vi "get_data_from_sensors.vi"() -> ()   [LabVIEW 2015]
uses:
  <vilib>/Analysis/baseanly.llb/Mean (DBL).vi
  <vilib>/ErrorRing/Error Ring.xnode
  <vilib>/Analysis/NI_AALBase.lvlib
panel:
  out "mean thermometer":dbl format="%0.2f"
  out "mean potentiometer":dbl format="%0.2f"
  out "min value potentiometer":sgl
  out "max value potentiometer":sgl
  out "min value thermometer":sgl
  out "max value thermometer":sgl
  out "Thermometer values":sgl[](array[numeric])
  out "Potentiometer values":sgl[](array[numeric])
  out "error out 3":errorcluster
  out "error out 2":errorcluster
  out "error out":errorcluster
  in  "stop":bool
  out "timed out?\nBattery Voltage\nPotentiometer":bool
  out "timed out?\nLink Quality\nPotentiometer":bool
  out "timed out?\nBattery Voltage\nTemperature":bool
  out "timed out?\nLink Quality\nTemperature":bool
  out "Link Quality\nTemperature (3212)":sgl
  out "Battery Voltage \nTemperature (3212)":sgl
  out "Link Quality\nPotentiometer (3202)":sgl
  out "Battery Voltage\nPotentiometer (3202)":sgl
  out "Waveform Chart":dbl(graph)
  out "Numeric":dbl
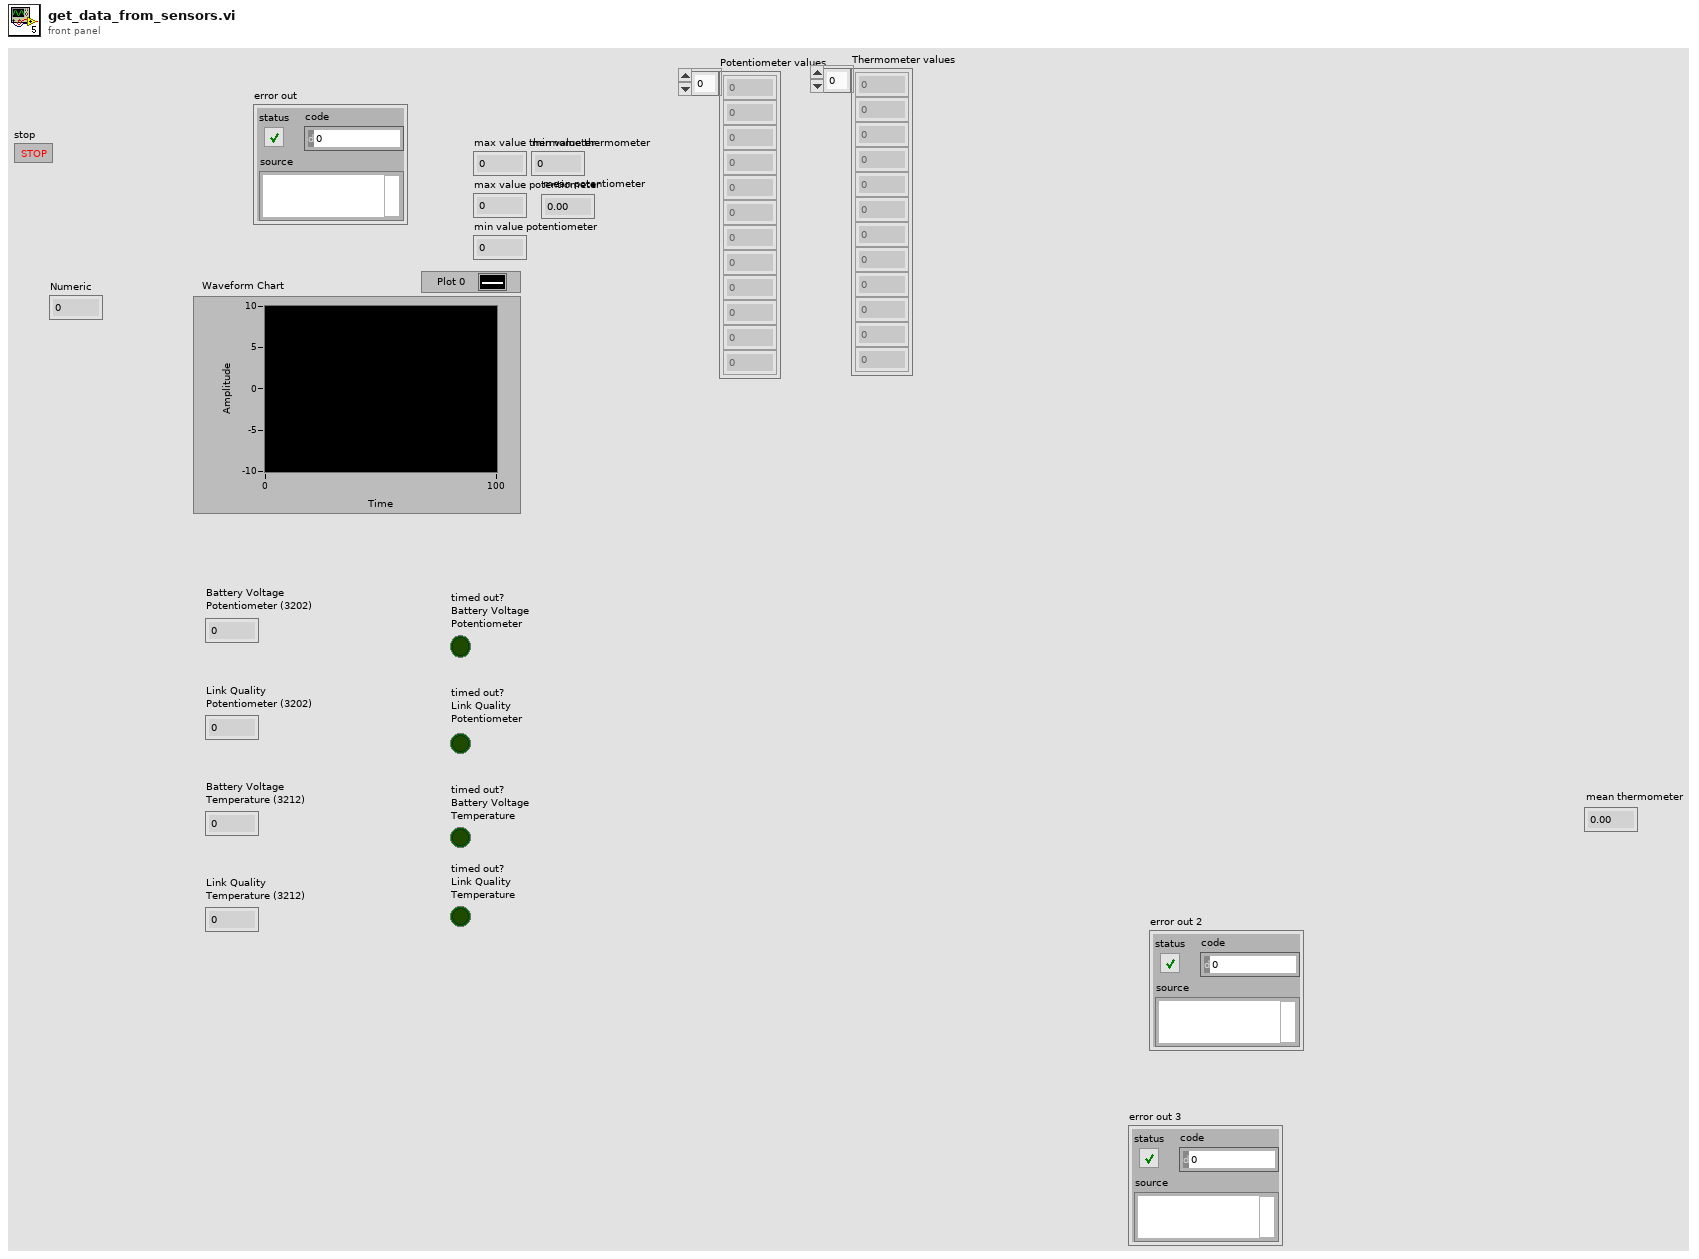
[diagram p1: front panel]
types:
  T1 = enum16{"open", "replace", "create", "open or create", "replace or create", "replace or create with confirmation"}
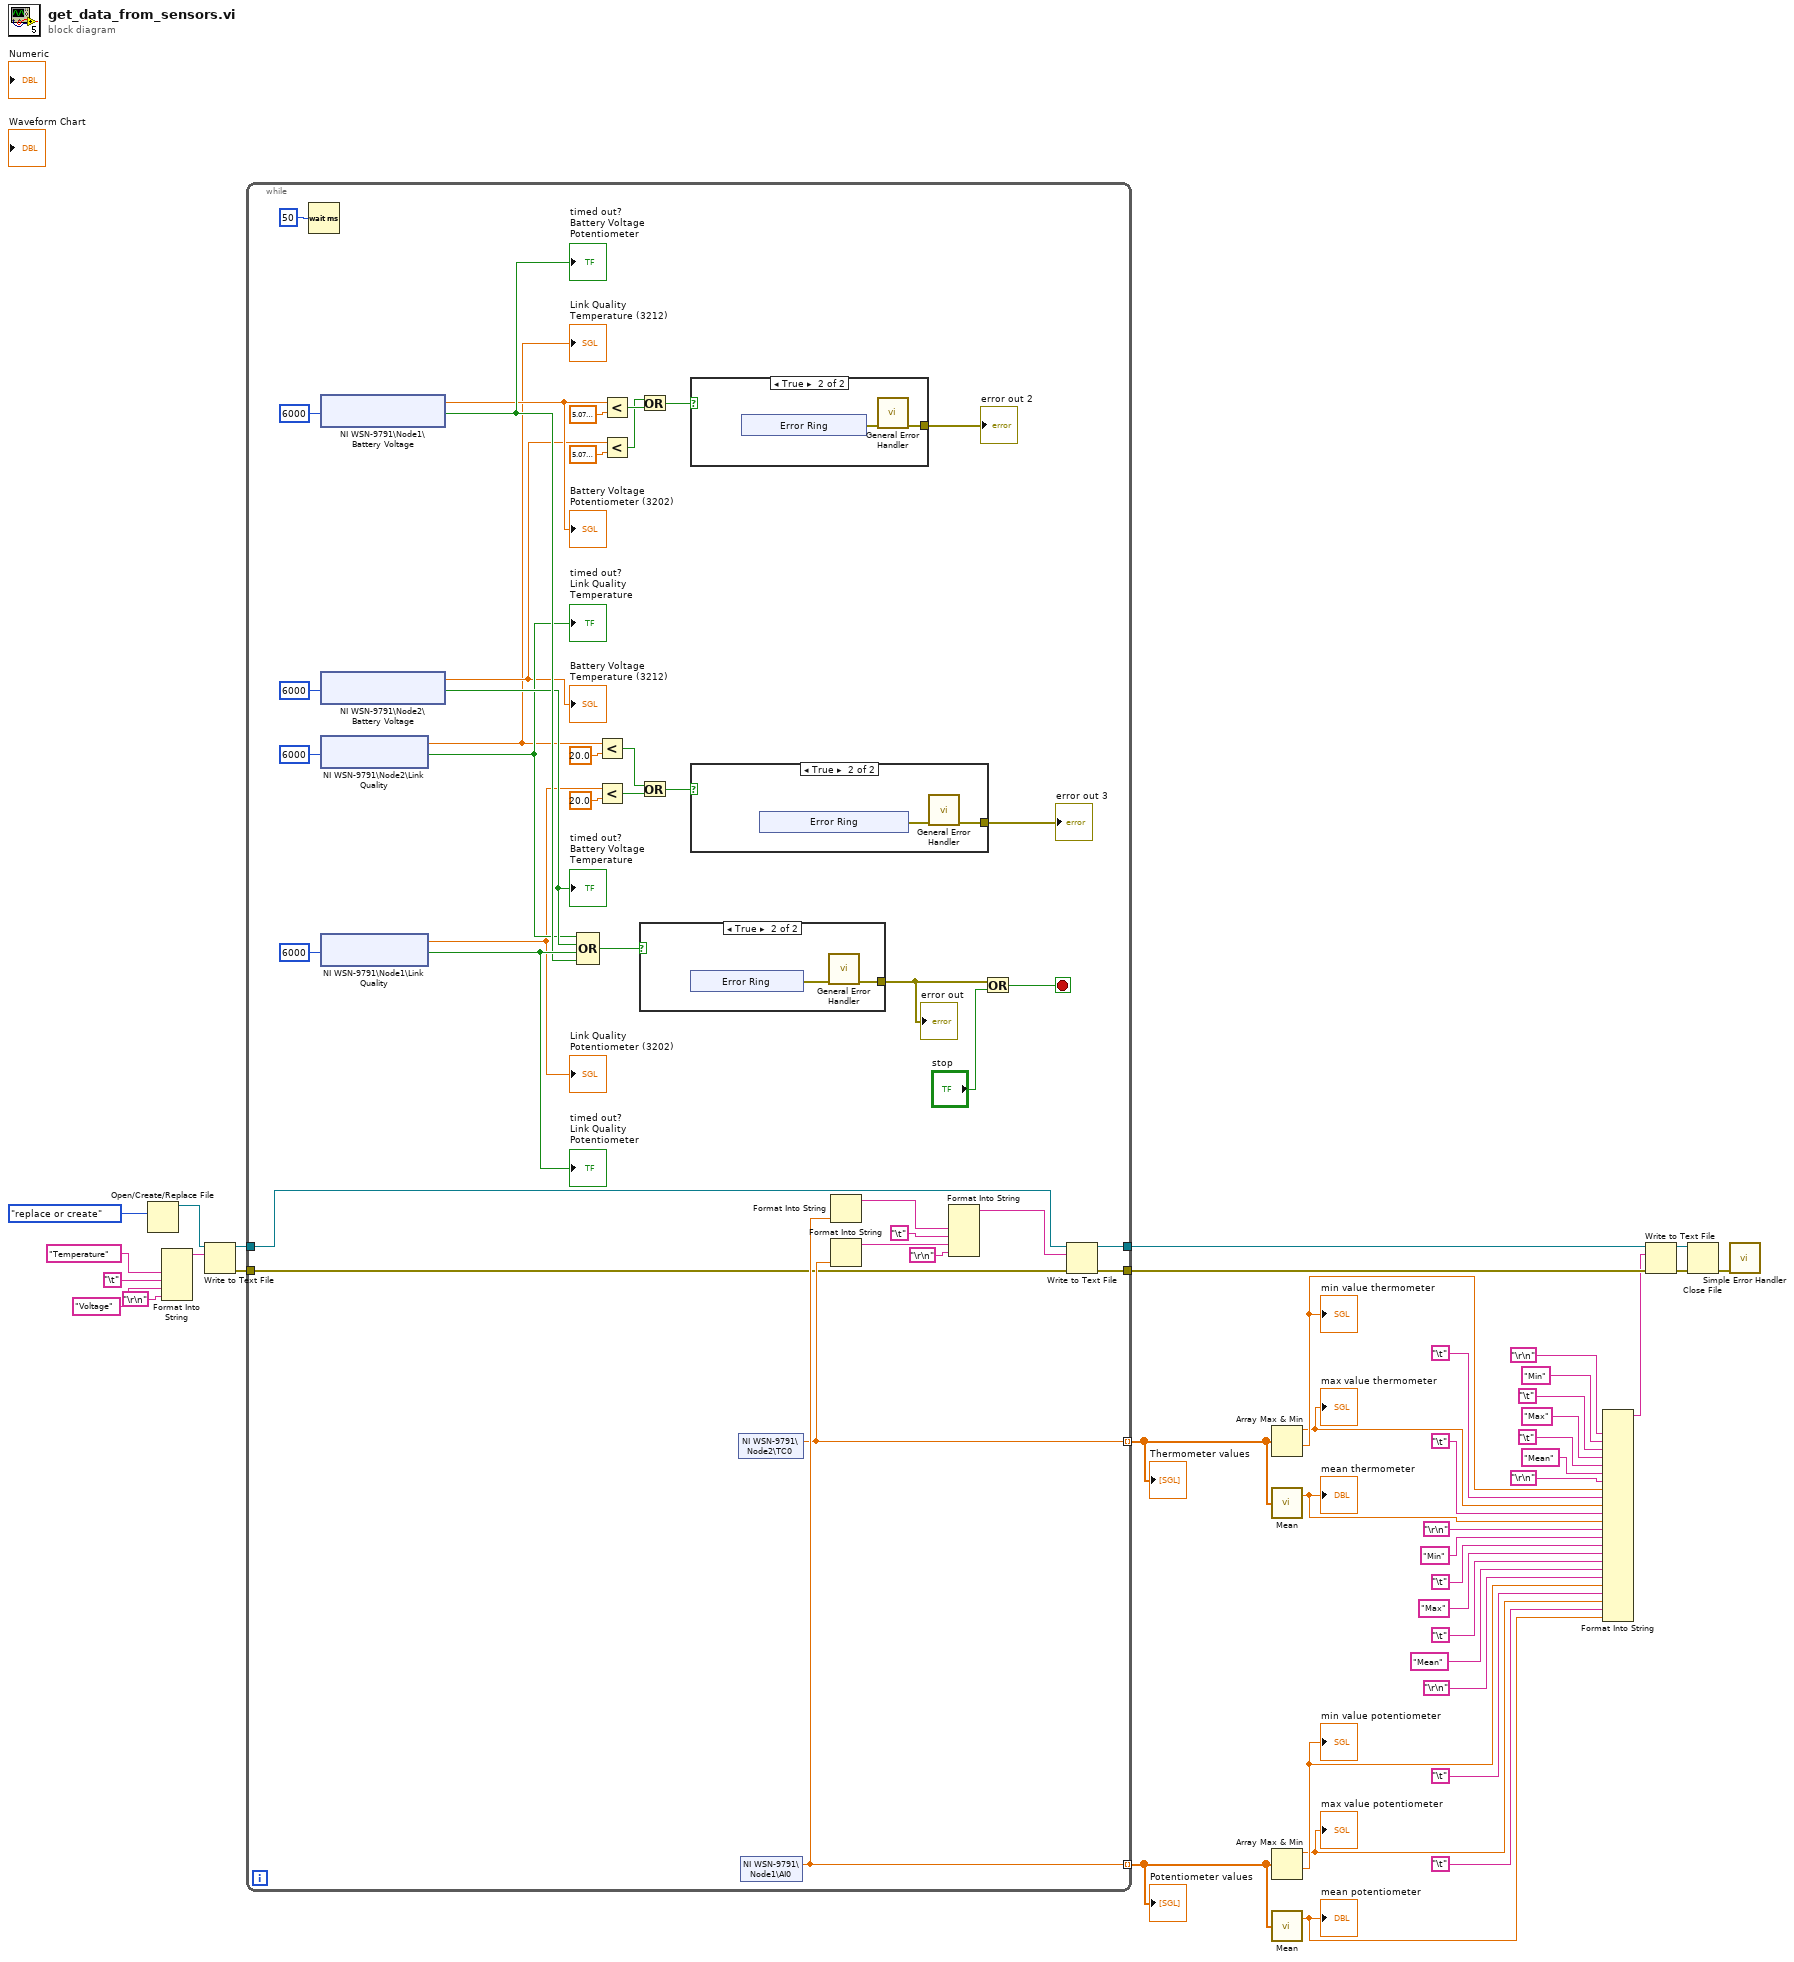
[diagram p0: block diagram]
diagram:
  n1 = Open/Create/Replace File(operation (0:open)=T1."replace or create") -> (refnum out=w33:refnum<file>)  [unwired: 5 in, 2 out]
  n2 = Format Into String("Temperature" ("input 1"), "\t", "Voltage" ("input 1"), "\r\n") -> (resulting string=w32:string)  [unwired: 3 in, 1 out]
  n3 = Write to Text File(file (use dialog)=w33, text=w32) -> (refnum out=w31:refnum<file>, error out=w30:errorcluster)  [unwired: 2 in, 1 out]
  n4 = while {
    tunnel: [w51] -> w40 mode=indexing
    tunnel: [w52] -> w41 mode=indexing
    tunnel: [w46] -> w27
    tunnel: [w45] -> w26
    tunnel: w31 -> [w43]
    tunnel: w30 -> [w42]
    stop <- w76 stop-if-true
    n5 = Wait (ms)(milliseconds to wait=u32 50) -> ()  [unwired: 1 out]
    n6 = shared-variable "NI WSN-9791\\Node1\\Battery Voltage"(6000 ("ms timeout (0)")) -> (w66:sgl, w72:bool)  [unwired: 1 in, 1 out]
    "Battery Voltage\nPotentiometer (3202)" <- w66
    "timed out?\nBattery Voltage\nPotentiometer" <- w72
    n7 = shared-variable "NI WSN-9791\\Node2\\Battery Voltage"(6000 ("ms timeout (0)")) -> (w62:sgl, w71:bool)  [unwired: 1 in, 1 out]
    "Battery Voltage \nTemperature (3212)" <- w62
    "timed out?\nBattery Voltage\nTemperature" <- w71
    n8 = shared-variable "NI WSN-9791\\Node2\\Link Quality"(6000 ("ms timeout (0)")) -> (w54:sgl, w70:bool)  [unwired: 1 in, 1 out]
    "Link Quality\nTemperature (3212)" <- w54
    "timed out?\nLink Quality\nTemperature" <- w70
    n9 = shared-variable "NI WSN-9791\\Node1\\Link Quality"(6000 ("ms timeout (0)")) -> (w58:sgl, w73:bool)  [unwired: 1 in, 1 out]
    "Link Quality\nPotentiometer (3202)" <- w58
    "timed out?\nLink Quality\nPotentiometer" <- w73
    n10 = Compound Arithmetic op=OR(w70, w71, w73, w72) -> (w69:bool)
    n11 = Less?(x=w54, y=sgl 20.0) -> (x < y?=w53:bool)
    n12 = Less?(x=w58, y=sgl 20.0) -> (x < y?=w56:bool)
    n13 = Less?(x=w66, y=sgl 5.08) -> (x < y?=w64:bool)
    n14 = Less?(x=w62, y=sgl 5.08) -> (x < y?=w61:bool)
    n15 = Or(x=w61, y=w64) -> (x .or. y?=w60:bool)
    n16 = Or(x=w53, y=w56) -> (x .or. y?=w57:bool)
    n17 = case shown="True" w69 {
      tunnel: [_ w89] -> w77
      frame False {
      }
      frame True {
        n18 = xnode "Error Ring"() -> ("error out"=w88:errorcluster)
        n19 = call <vilib>:"General Error Handler.vi"("error in (no error)"=w88) -> ("error out"=w89:errorcluster)  [unwired: 10 in, 4 out]
      }
    }
    "error out" <- w77
    n20 = case shown="True" w60 {
      tunnel: [_ w86] -> w68
      frame False {
      }
      frame True {
        n21 = xnode "Error Ring"() -> ("error out"=w85:errorcluster)
        n22 = call <vilib>:"General Error Handler.vi"("error in (no error)"=w85) -> ("error out"=w86:errorcluster)  [unwired: 10 in, 4 out]
      }
    }
    "error out 2" <- w68
    n23 = case shown="True" w57 {
      tunnel: [_ w83] -> w67
      frame False {
      }
      frame True {
        n24 = xnode "Error Ring"() -> ("error out"=w82:errorcluster)
        n25 = call <vilib>:"General Error Handler.vi"("error in (no error)"=w82) -> ("error out"=w83:errorcluster)  [unwired: 10 in, 4 out]
      }
    }
    "error out 3" <- w67
    n26 = shared-variable "NI WSN-9791\\Node2\\TC0"() -> (w51:sgl)  [unwired: 1 in, 1 out]
    n27 = shared-variable "NI WSN-9791\\Node1\\AI0"() -> (w52:sgl)  [unwired: 1 in, 1 out]
    n28 = Format Into String(w52) -> (resulting string=w50:string)  [unwired: 3 in, 1 out]
    n29 = Format Into String(w51) -> (resulting string=w48:string)  [unwired: 3 in, 1 out]
    n30 = Format Into String(w50, "\t", w48, "\r\n") -> (resulting string=w47:string)  [unwired: 3 in, 1 out]
    n31 = Or(x=w77, y="stop") -> (x .or. y?=w76:bool)
    n32 = Write to Text File(file (use dialog)=w43, text=w47, error in=w42) -> (refnum out=w46:refnum<file>, error out=w45:errorcluster)  [unwired: 1 in, 1 out]
  }
  "Potentiometer values" <- w41
  "Thermometer values" <- w40
  n33 = Array Max & Min(array=w40) -> (max value=w16:sgl, min value=w17:sgl)  [unwired: 2 out]
  "max value thermometer" <- w16
  "min value thermometer" <- w17
  n34 = call-poly <vilib>:"Mean.vi"("X"=w40) -> ("mean"=w15:dbl)  [unwired: 1 out]
  "mean thermometer" <- w15
  n35 = Array Max & Min(array=w41) -> (max value=w4:sgl, min value=w5:sgl)  [unwired: 2 out]
  "max value potentiometer" <- w4
  "min value potentiometer" <- w5
  n36 = call-poly <vilib>:"Mean.vi"("X"=w41) -> ("mean"=w3:dbl)  [unwired: 1 out]
  "mean potentiometer" <- w3
  n37 = Format Into String("\r\n", "Min" ("input 1"), "\t", "Max" ("input 1"), "\t", "Mean" ("input 1"), "\r\n", w17, "\t", w16, "\t", w15, "\r\n", "Min" ("input 1"), "\t", "Max" ("input 1"), "\t", "Mean" ("input 1"), "\r\n", w5, "\t", w4, "\t", w3) -> (resulting string=w18:string)  [unwired: 3 in, 1 out]
  n38 = Write to Text File(file (use dialog)=w27, text=w18, error in=w26) -> (refnum out=w29:refnum<file>, error out=w28:errorcluster)  [unwired: 1 in, 1 out]
  n39 = Close File(refnum=w29, error in=w28) -> (error out=w38:errorcluster)  [unwired: 1 out]
  n40 = call <vilib>:"Simple Error Handler.vi"("error in (no error)"=w38) -> ()  [unwired: 4 in, 5 out]
